vi "ex11.vi"() -> ()   [LabVIEW 2019]
panel:
  out "数値表示器":dbl
  in  "数値制御器":dbl
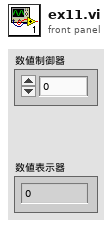
[diagram p1: front panel]
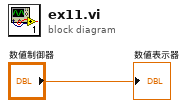
[diagram p0: block diagram]
diagram:
  "数値表示器" <- "数値制御器"
